vi "CopyClearTempImage.vi"(8 "error in (no error)":errorcluster, 10 "Display Image In":T1, 11 "TempImageRefIn":T1) -> (0 "error out":errorcluster, 3 "DisplayImageOut":T1)   [LabVIEW 2019]
uses:
  <vilib>/vision/Image Controls.llb/IMAQ Image.ctl
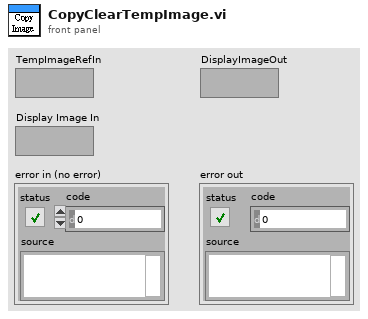
[diagram p1: front panel]
types:
  T1 = typedef "IMAQ Image.ctl" = refnum<image>
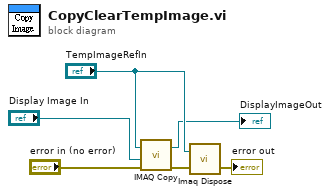
[diagram p0: block diagram]
diagram:
  n1 = call "IMAQ Copy"("error in (no error)"="error in (no error)", "Image Dst"="Display Image In", "Image Src"="TempImageRefIn") -> ("error out"=w1:errorcluster, "Image Dst Out"=→"DisplayImageOut":T1)  [unwired: 3 in]
  n2 = call "Imaq Dispose"("Image"="TempImageRefIn", "error in (no error)"=w1) -> ("error out"=→"error out":errorcluster)  [unwired: 4 in]
